vi "from string 3.0.vi"(8 "error in":errorcluster, 10 "data in":string, 11 "Shared Memory configuration in":refnum<class "Shared Memory configuration.lvclass">) -> (0 "error out":errorcluster, 2 "remaining data":string, 3 "Shared Memory configuration out":refnum<class "Shared Memory configuration.lvclass">)   [LabVIEW 2013, in "Shared Memory configuration.lvclass"]
uses:
  Shared Memory configuration.lvclass
  editor node/sync/sync item.ctl
  editor node/sync/sync mechanism.ctl
  Shared Memory configuration.lvclass/Shared Memory configuration.ctl
  <vilib>/NI/Configuration Framework/serializable configuration/NISE_CEF_serializable configuration.lvclass
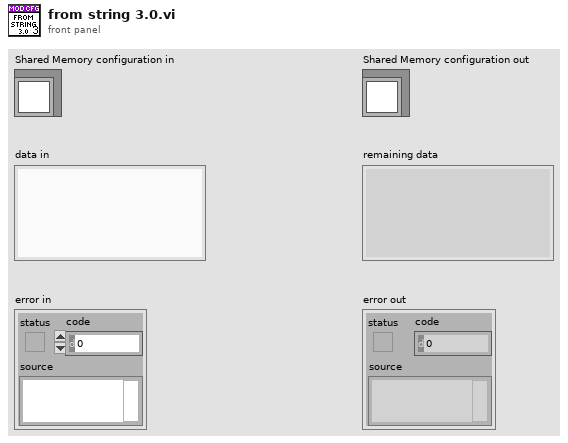
[diagram p1: front panel]
types:
  T1 = typedef "Shared Memory configuration.lvclass/sync item.ctl" = cluster{"mechanism":T2, "name":string}
  T2 = typedef "Shared Memory configuration.lvclass/sync mechanism.ctl" = enum16{"Semaphore"}
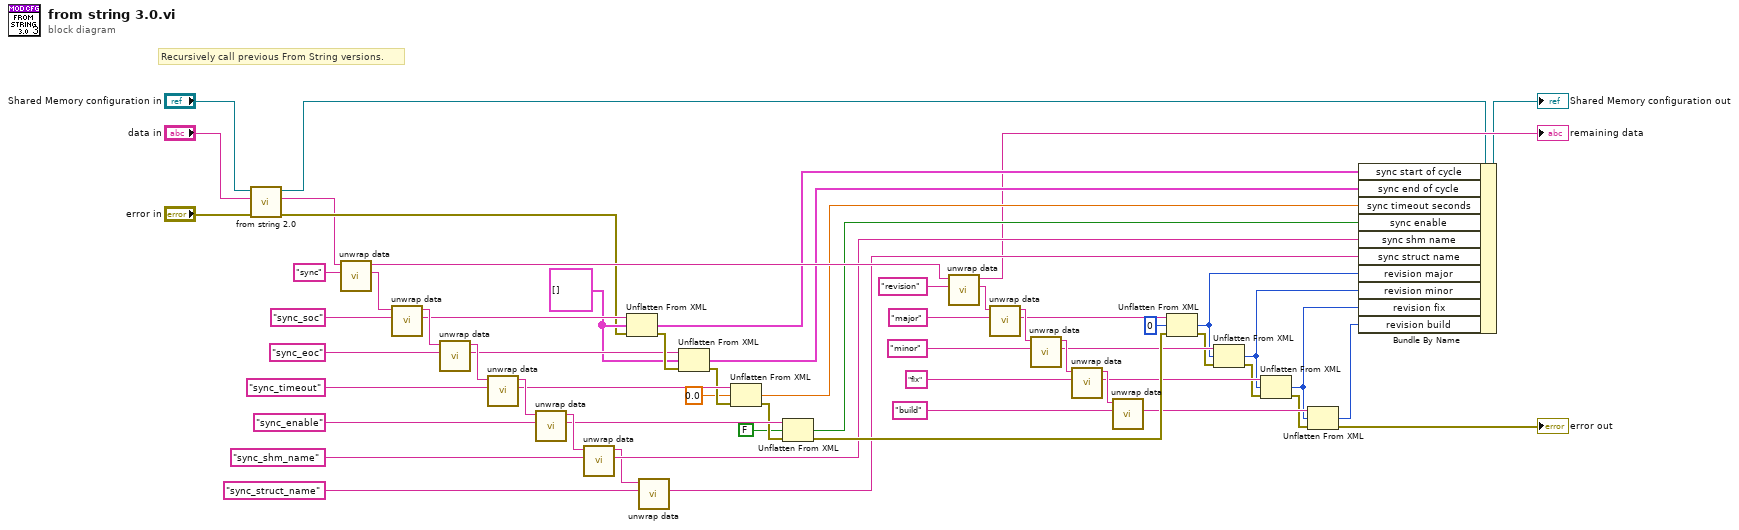
[diagram p0: block diagram]
diagram:
  w42 = T1[] [] ("sync start of cycle")
  # "Recursively call previous From String versions."
  n1 = call "from string 2.0.vi"("error in"="error in", "data in"="data in", "Shared Memory configuration in"="Shared Memory configuration in") -> ("error out"=w5:errorcluster, "remaining data"=w4:string, "Shared Memory configuration out"=w2:refnum<class "Shared Memory configuration.lvclass">)  [unwired: 6 in]
  n2 = call <vilib>:"unwrap data.vi"("identifier"="sync", "data to unwrap"=w4) -> ("unwrapped data"=w48:string, "remaining string"=w54:string)  [unwired: 8 in]
  n3 = call <vilib>:"unwrap data.vi"("identifier"="sync_soc", "data to unwrap"=w48) -> ("unwrapped data"=w44:string, "remaining string"=w47:string)  [unwired: 8 in]
  n4 = call <vilib>:"unwrap data.vi"("identifier"="sync_eoc", "data to unwrap"=w47) -> ("unwrapped data"=w43:string, "remaining string"=w46:string)  [unwired: 8 in]
  n5 = call <vilib>:"unwrap data.vi"("identifier"="sync_timeout", "data to unwrap"=w46) -> ("unwrapped data"=w41:string, "remaining string"=w45:string)  [unwired: 8 in]
  n6 = call <vilib>:"unwrap data.vi"("identifier"="sync_enable", "data to unwrap"=w45) -> ("unwrapped data"=w39:string, "remaining string"=w40:string)  [unwired: 8 in]
  n7 = call <vilib>:"unwrap data.vi"("identifier"="sync_shm_name", "data to unwrap"=w40) -> ("unwrapped data"=w30:string, "remaining string"=w8:string)  [unwired: 8 in]
  n8 = Unflatten From XML(xml string=w44, type=w42, error in (no error)=w5) -> (value=w34:T1[], error out=w57:errorcluster)
  n9 = call <vilib>:"unwrap data.vi"("identifier"="sync_struct_name", "data to unwrap"=w8) -> ("unwrapped data"=w7:string)  [unwired: 8 in, 1 out]
  n10 = Unflatten From XML(xml string=w43, type=w42, error in (no error)=w57) -> (value=w33:T1[], error out=w38:errorcluster)
  n11 = Unflatten From XML(xml string=w41, type=0.0, error in (no error)=w38) -> (value=w32:dbl, error out=w37:errorcluster)
  n12 = Unflatten From XML(xml string=w39, type=FALSE, error in (no error)=w37) -> (value=w31:bool, error out=w58:errorcluster)
  n13 = call <vilib>:"unwrap data.vi"("identifier"="revision", "data to unwrap"=w54) -> ("unwrapped data"=w10:string, "remaining string"=→"remaining data":string)  [unwired: 8 in]
  n14 = call <vilib>:"unwrap data.vi"("identifier"="major", "data to unwrap"=w10) -> ("unwrapped data"=w23:string, "remaining string"=w29:string)  [unwired: 8 in]
  n15 = call <vilib>:"unwrap data.vi"("identifier"="minor", "data to unwrap"=w29) -> ("unwrapped data"=w24:string, "remaining string"=w28:string)  [unwired: 8 in]
  n16 = call <vilib>:"unwrap data.vi"("identifier"="fix", "data to unwrap"=w28) -> ("unwrapped data"=w25:string, "remaining string"=w27:string)  [unwired: 8 in]
  n17 = call <vilib>:"unwrap data.vi"("identifier"="build", "data to unwrap"=w27) -> ("unwrapped data"=w26:string)  [unwired: 8 in, 1 out]
  n18 = Unflatten From XML(xml string=w23, type=u8 0, error in (no error)=w58) -> (value=w14:u8, error out=w18:errorcluster)
  n19 = Unflatten From XML(xml string=w24, type=w14, error in (no error)=w18) -> (value=w13:u8, error out=w17:errorcluster)
  n20 = Unflatten From XML(xml string=w25, type=w13, error in (no error)=w17) -> (value=w12:u8, error out=w16:errorcluster)
  n21 = Unflatten From XML(xml string=w26, type=w12, error in (no error)=w16) -> (value=w11:u8, error out=→"error out":errorcluster)
  n22 = Bundle By Name(cluster=w2, "sync start of cycle"=w34, "sync end of cycle"=w33, "sync timeout seconds"=w32, "sync enable"=w31, "sync shm name"=w30, "sync struct name"=w7, "revision major"=w14, "revision minor"=w13, "revision fix"=w12, "revision build"=w11) -> (→"Shared Memory configuration out":refnum<class "Shared Memory configuration.lvclass">)
